vi "Return Primary String Numeric (SubVI).vi"(7 "String-DBL Control":T1, 8 "error in":errorcluster, 11 "Primary Numeric":dbl) -> (0 "error out":errorcluster, 2 "Primary String":string, 3 "Primary Numeric":dbl format="%#_8g")   [LabVIEW 2021]
doc: "This VI performs String-DBL and DBL-String conversion, depending on the value of the command."
uses:
  Controls/String-Double Conversion Control.ctl
  Controls/String Commands.ctl
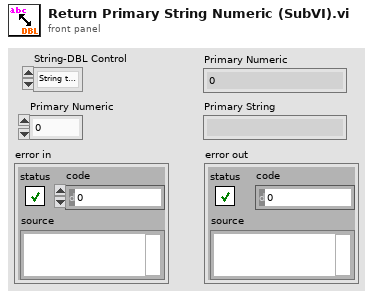
[diagram p1: front panel]
types:
  T1 = typedef "String-Double Conversion Control.ctl" = enum16{"String to DBL", "DBL to String"}
  T2 = typedef "String Commands.ctl" = enum16{"GET Strings", "Set Secondary", "Build Primary", "Build Secondary", "Backspace", "Replace Operator", "Clear Primary", "Clear Secondary", "Clear ALL", "Decimal Point"}
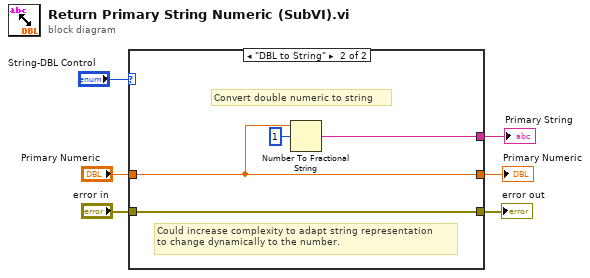
[diagram p0: block diagram]
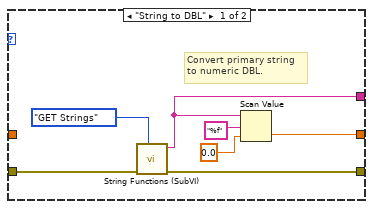
[diagram p2: hidden frame]
diagram:
  n1 = case shown="\"DBL to String\"" "String-DBL Control" {
    tunnel: "error in" -> [w13 w17]
    tunnel: [w9 w16] -> w5
    tunnel: [w8 w17] -> w4
    tunnel: "Primary Numeric" -> [_ w16]
    tunnel: [w7 w15] -> w1
    frame "String to DBL" {
      # "Convert primary string\nto numeric DBL."
      n2 = call "String Functions (SubVI).vi"("String Function"=String_Commands."GET Strings", "error in"=w13) -> ("error out"=w8:errorcluster, "Primary Display String"=w7:string)  [unwired: 7 in, 1 out]
      n3 = Scan Value(string=w7, format string="%f", default (0 dbl)=0.0) -> (value=w9:dbl)  [unwired: 1 out]
    }
    frame "DBL to String" {
      # "Could increase complexity to adapt string representation\nto change dynamically to the number."
      # "Convert double numeric to string"
      n4 = Number To Fractional String(number=w16, width (-)=i16 1) -> (F-format string=w15:string)  [unwired: 2 in]
    }
  }
  "error out" <- w4
  "Primary Numeric" <- w5
  "Primary String" <- w1
